vi "SVM Train NU_SVC.vi"(7 "Options":T9={"cache_size"=200.0, "eps"=0.001, "shrinking"=TRUE, "probability"=FALSE}, 8 "error in (no error)":errorcluster, 9 "nu":T1=0.5 caption="nu (0,5)", 10 "Kernel":T8, 11 "Problem":T7) -> (0 "error out":errorcluster, 3 "Model":T2)   [LabVIEW 2014]
doc: "This function constructs and returns an SVM model according to the given training data and parameters.\n\nThe parameter nu controls the number of support vectors and training errors. It specifies an upper bound on the fraction of training errors and a lower bound of the fraction of support vectors. It needs to be in the range (0,1].\n\nIt can be shown that the nu-SVC formulation is a reparametrization of the C-SVC and therefore mathematically equivalent (ref: scikit-learn documentation)."
uses:
  Controls/Options Training.ctl
  Controls/Kernel.ctl
  Libsvm Wrapper/Controls/svm_kernel_type.ctl
  Libsvm Wrapper/Controls/svm_problem.ctl
  Libsvm Wrapper/Controls/svm_node.ctl
  Libsvm Wrapper/Controls/svm_model.ctl
  Libsvm Wrapper/Controls/svm_parameter.ctl
  Libsvm Wrapper/Controls/svm_type.ctl
  Controls/Parameters NU_SVC.ctl
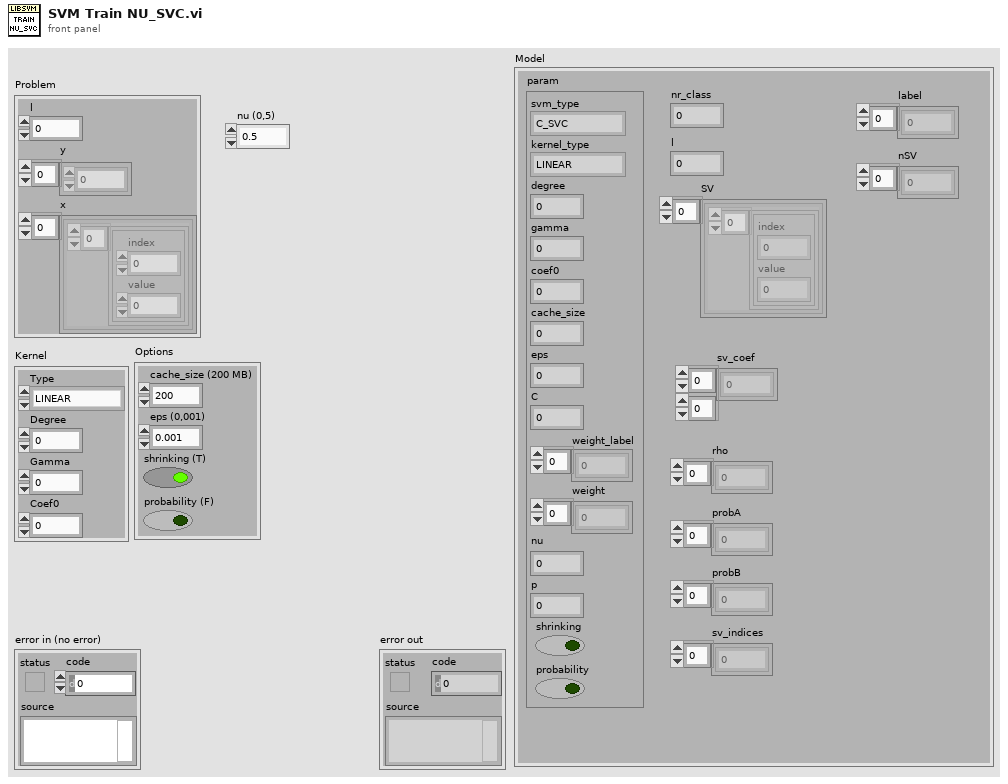
[diagram p1: front panel]
types:
  T1 = typedef "Parameters NU_SVC.ctl" = dbl
  T2 = typedef "svm_model.ctl" = cluster{"param":T3, "nr_class":i32, "l":i32, "SV":cluster{"Array":T6[]}[], "sv_coef":dbl[][], "rho":dbl[], "probA":dbl[], "probB":dbl[], "sv_indices":i32[], "label":i32[], "nSV":i32[]}
  T3 = typedef "svm_parameter.ctl" = cluster{"svm_type":T4, "kernel_type":T5, "degree":i32, "gamma":dbl, "coef0":dbl, "cache_size":dbl, "eps":dbl, "C":dbl, "weight_label":i32[], "weight":dbl[], "nu":dbl, "p":dbl, "shrinking":bool, "probability":bool}
  T4 = typedef "svm_type.ctl" = enum32{"C_SVC", "NU_SVC", "ONE_CLASS", "EPSILON_SVR", "NU_SVR"}
  T5 = typedef "svm_kernel_type.ctl" = enum32{"LINEAR", "POLY", "RBF", "SIGMOID", "PRECOMPUTED"}
  T6 = typedef "svm_node.ctl" = cluster{"index":i32, "value":dbl}
  T7 = typedef "svm_problem.ctl" = cluster{"l":i32, "y":dbl[], "x":cluster{T6[]}[]}
  T8 = typedef "Kernel.ctl" = cluster{"Type":T5, "Degree":i32, "Gamma":dbl, "Coef0":dbl}
  T9 = typedef "Options Training.ctl" = cluster{"cache_size":dbl, "eps":dbl, "shrinking":bool, "probability":bool}
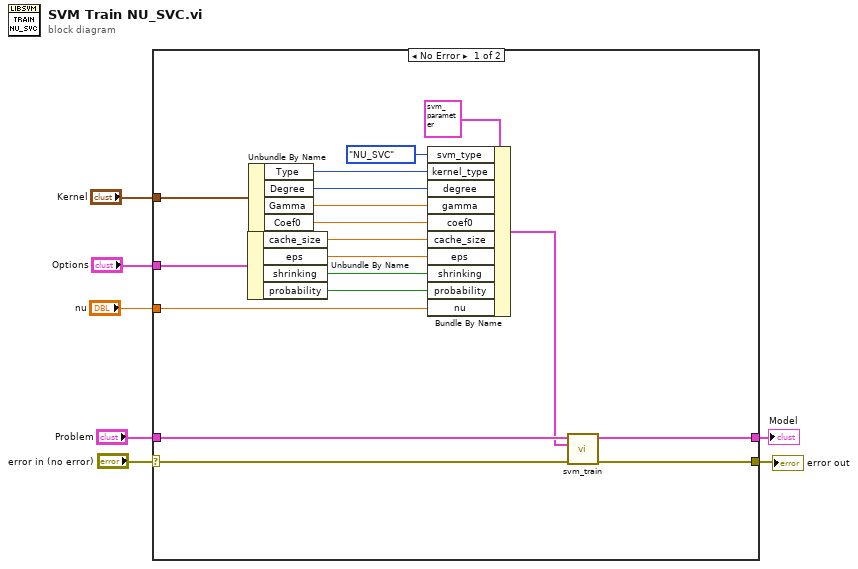
[diagram p0: block diagram]
diagram:
  n1 = case shown="No Error" "error in (no error)" {
    selector: "error in (no error)" -> [w25 w26]
    tunnel: [w24 w26] -> w7
    tunnel: "Problem" -> [w22 _]
    tunnel: "Kernel" -> [w21 _]
    tunnel: [w14 _] -> w3
    tunnel: "Options" -> [w11 _]
    tunnel: "nu" -> [w8 _]
    frame No Error {
      n2 = Unbundle By Name(w11) -> ("cache_size"=w13:dbl, "eps"=w12:dbl, "shrinking"=w10:bool, "probability"=w9:bool)
      n3 = Unbundle By Name(w21) -> ("Type"=w20:T5, "Degree"=w19:i32, "Gamma"=w18:dbl, "Coef0"=w17:dbl)
      n4 = Bundle By Name(cluster=T3 {"svm_type"=enum."C_SVC", "kernel_type"=enum."LINEAR", "degree"=0, "gamma"=0.0, "coef0"=0.0, "cache_size"=0.0, "eps"=0.0, "C"=0.0, "weight_label"=[], "weight"=[], "nu"=0.0, "p"=0.0, "shrinking"=FALSE, "probability"=FALSE} ("svm_parameter"), "svm_type"=svm_type."NU_SVC", "kernel_type"=w20, "degree"=w19, "gamma"=w18, "coef0"=w17, "cache_size"=w13, "eps"=w12, "shrinking"=w10, "probability"=w9, "nu"=w8) -> (w15:T3)
      n5 = call "svm_train.vi"("error in (no error)"=w25, "Parameters"=w15, "Problem"=w22) -> ("error out"=w24:errorcluster, "Model"=w14:T2)  [unwired: 7 in]
    }
    frame Error {
    }
  }
  "error out" <- w7
  "Model" <- w3
